vi "write system session.vi"(8 "error in":errorcluster, 10 "system session":refnum<data-value>, 11 "SysCfg Device in":refnum<class "SysCfg Device.lvclass">) -> (0 "error out":errorcluster, 3 "SysCfg Device out":refnum<class "SysCfg Device.lvclass">)   [LabVIEW 2016, in "SMI.lvlib" / "SysCfg Device.lvclass"]
uses:
  SysCfg Device.lvclass
  SysCfg Device.lvclass/SysCfg Device.ctl
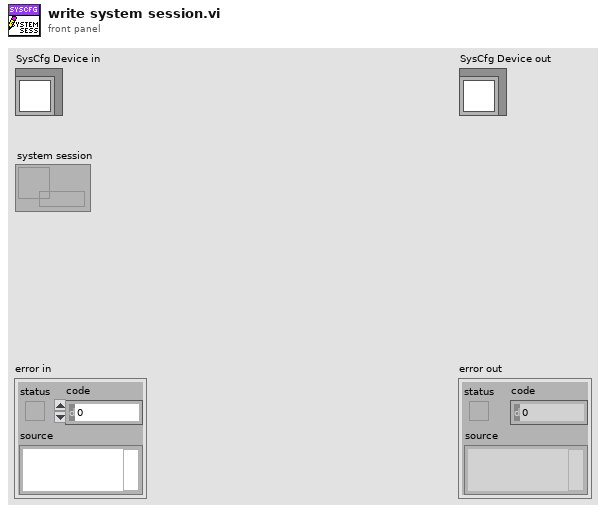
[diagram p1: front panel]
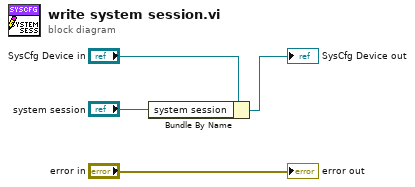
[diagram p0: block diagram]
diagram:
  n1 = Bundle By Name(cluster="SysCfg Device in", "system session"="system session") -> (→"SysCfg Device out":refnum<class "SysCfg Device.lvclass">)
  "error out" <- "error in"
